vi "save_config_v4.vi"(0 "Refnum VISA en entrée":refnum<visa-resource-name>, 1 "EXPT":dbl, 2 "Nstart_laser":u32, 3 "config Name":string, 4 "BETWEEN_PAT":u32, 5 "BIN":u16, 6 "NPAT":u32, 8 "Non_laser":u32, 9 "ROMODE":u32, 10 "SOFT_VERSION":string, 11 "Camera infos":string, 12 "Noff_laser":u32, 14 "Config Directory":path, 16 "USED_FILTERS":u8[](array[numeric]), 17 "STAGE_SPEED":dbl, 18 "USED_LEDS":bool[][](array[boolean]), 19 "XYPOS":T1, 26 "BETWEEN_SCAN":u32, 27 "NSCAN":u32) -> ()   [LabVIEW 2013]
uses:
  <vilib>/Analysis/Matrix/Datatypes/RealMatrix.ctl
  <vilib>/Analysis/Matrix/NI_Matrix.lvlib
panel:
  in  "Nstart_fluidics":u32
  in  "Non_fluidics":u32
  in  "Noff_fluidics":u32
  in  "SHOOT duration":dbl
  in  "shoot_at_SCAN":u32
  in  "useFLUIDICS":bool
  in  "isSINGLEshoot":bool
  in  "useLASER":bool
  in  "MIN. SCAN duration":dbl
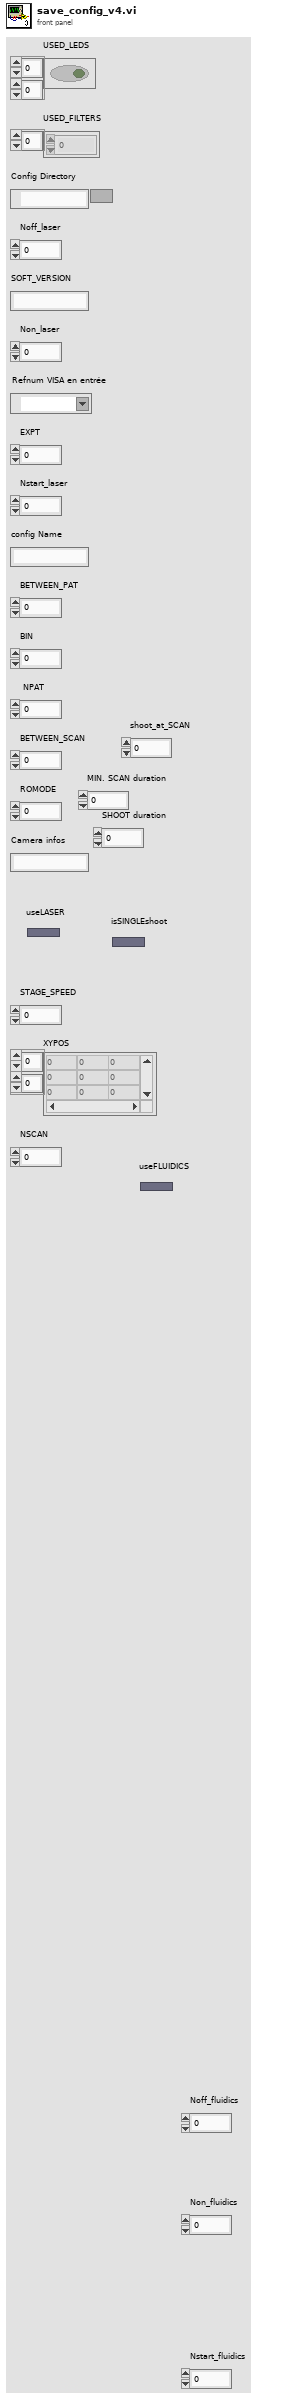
[diagram p1: front panel]
types:
  T1 = typedef "NI_Matrix.lvlib/RealMatrix.ctl" = dbl[][]
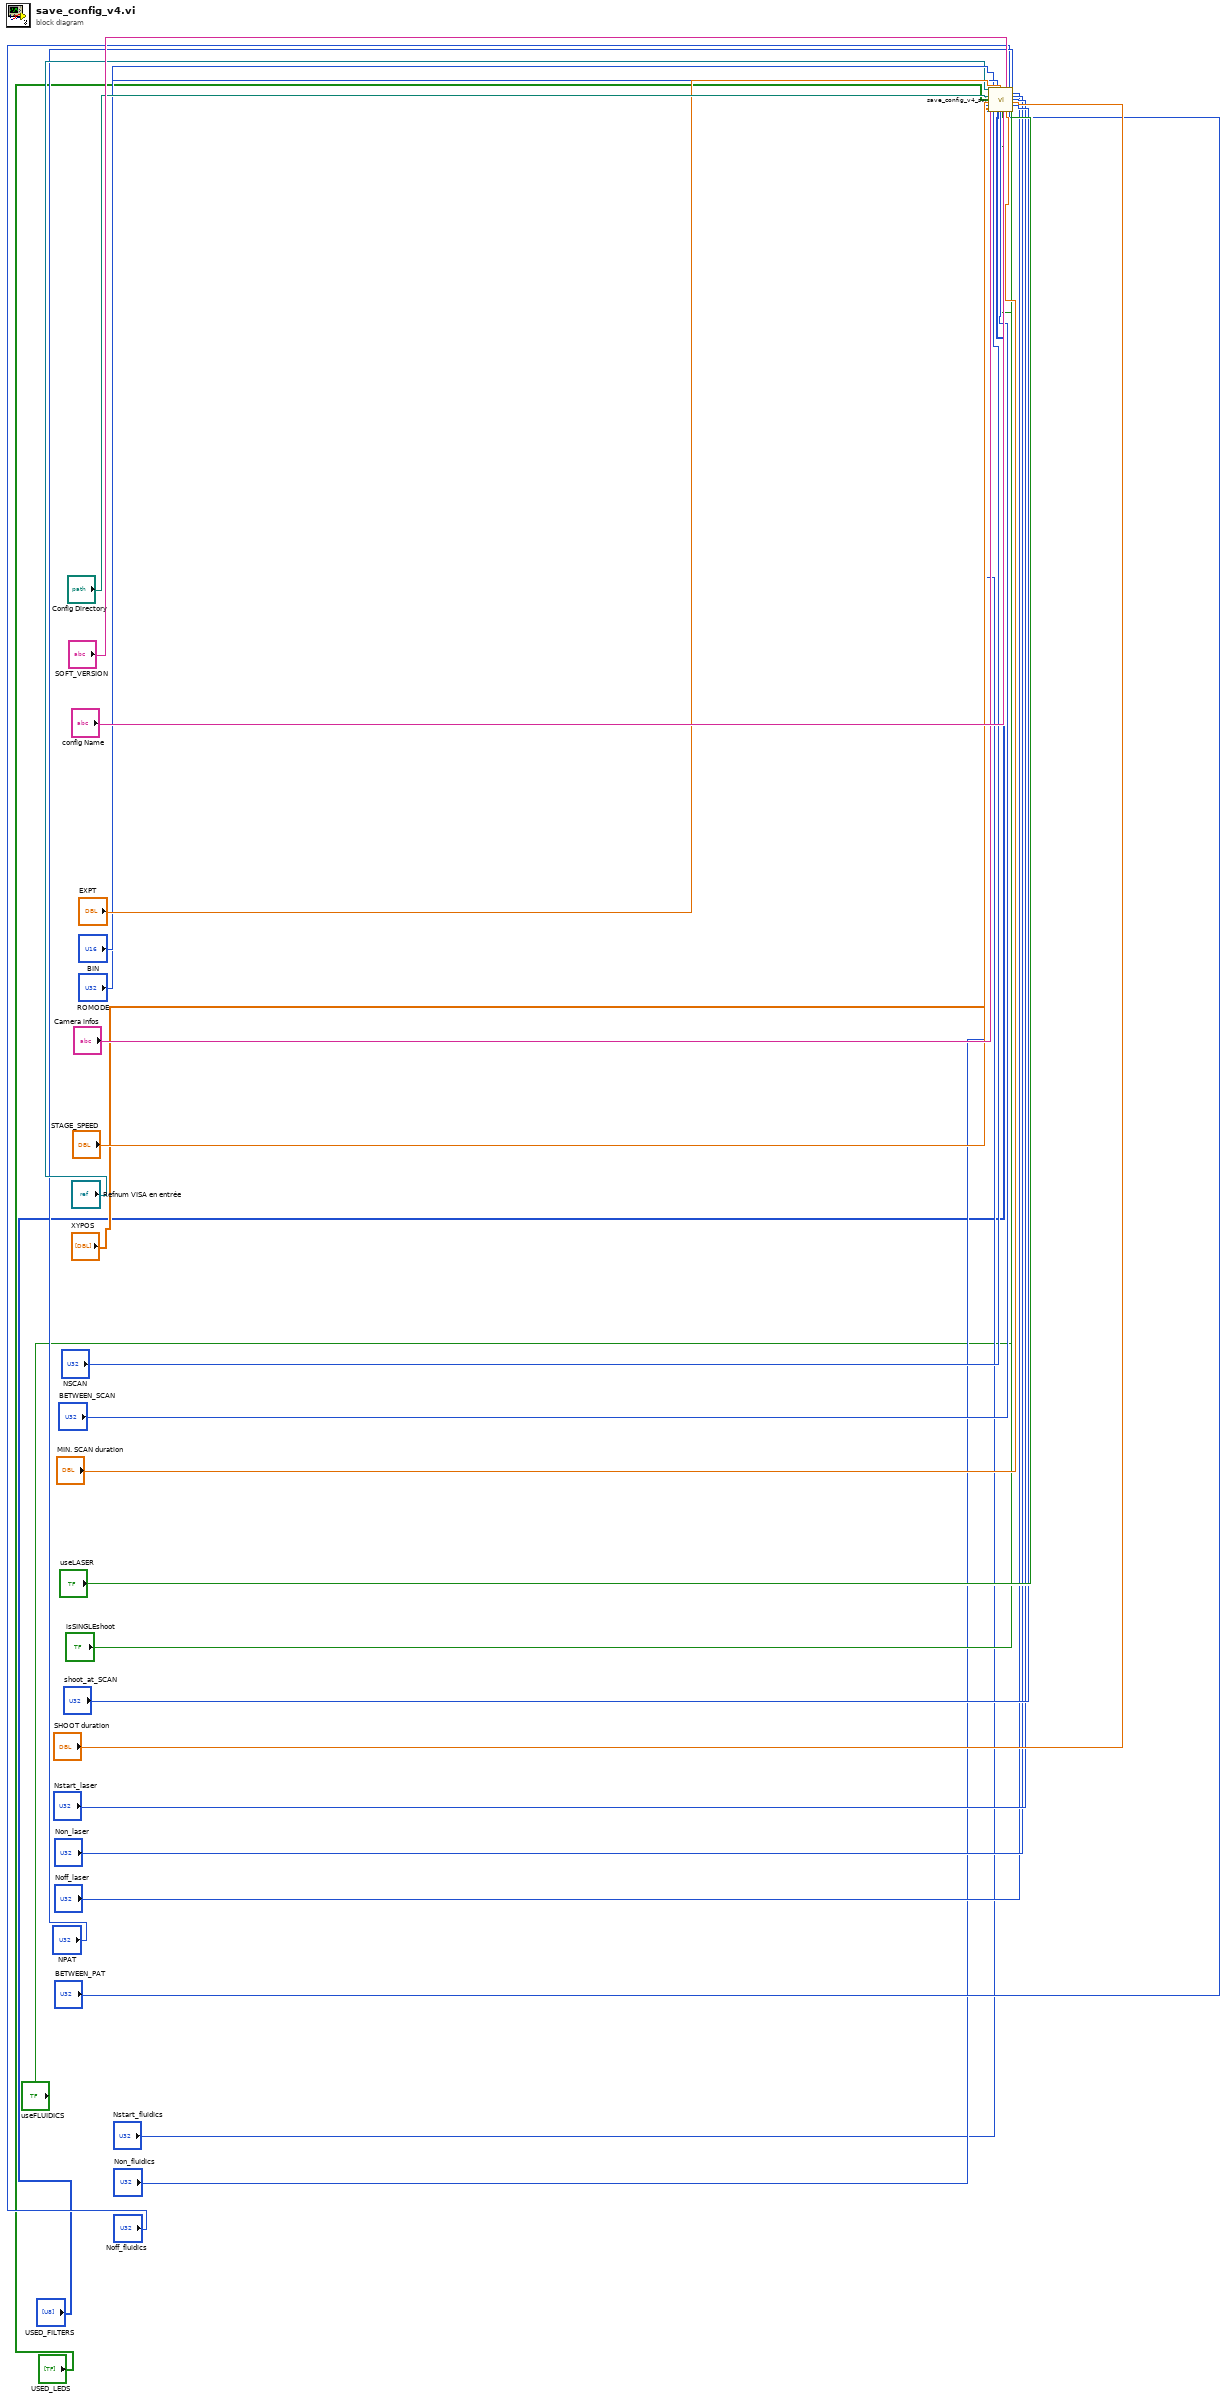
[diagram p0: block diagram]
diagram:
  n1 = call "save_config_v4_svi.vi"("Refnum VISA en entrée"="Refnum VISA en entrée", "Camera infos"="Camera infos", "Config Directory"="Config Directory", "USED_LEDS"="USED_LEDS", "STAGE_SPEED"="STAGE_SPEED", "Non_fluidics"="Non_fluidics", "XYPOS"="XYPOS", "Nstart_fluidics"="Nstart_fluidics", "ROMODE"="ROMODE", "NSCAN"="NSCAN", "BIN"="BIN", "USED_FILTERS"="USED_FILTERS", "EXPT"="EXPT", "BETWEEN_SCAN"="BETWEEN_SCAN", "config Name"="config Name", "useFLUIDICS"="useFLUIDICS", "SOFT_VERSION"="SOFT_VERSION", "MIN. SCAN duration"="MIN. SCAN duration", "Noff_fluidics"="Noff_fluidics", "BETWEEN_PAT"="BETWEEN_PAT", "NPAT"="NPAT", "Noff_laser"="Noff_laser", "Non_laser"="Non_laser", "Nstart_laser"="Nstart_laser", "SHOOT duration"="SHOOT duration", "shoot_at_SCAN"="shoot_at_SCAN", "isSINGLEshoot"="isSINGLEshoot", "useLASER"="useLASER") -> ()
